vi "DAQ_SampleLoop.vi"(0 "reference in":refnum<class "NI_DAQ.lvclass">, 5 "error in (no error)":errorcluster) -> (14 "reference out":refnum<class "NI_DAQ.lvclass">, 15 "RealTimeValue":dbl[](array[numeric]), 19 "error out":errorcluster)   [LabVIEW 2020, in "DAQ.lvlib" / "NI_DAQ.lvclass"]
uses:
  NI_DAQ.lvclass
  D:/BingoGithub/DAQ_V000.04/DAQ_Module/DAQ_Base_class/DAQ_Base.lvclass
  DAQ_Base_class/DAQ_Base.lvclass
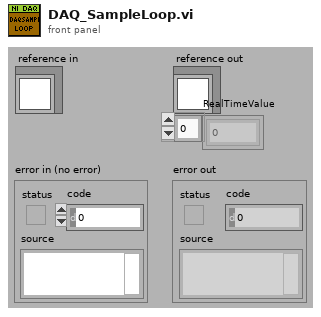
[diagram p1: front panel]
types:
  T1 = typedef "DAQ.lvlib/DAQ_Base.lvclass/ObjectAttributesRef.ctl" = refnum<data-value>
  T2 = typedef "DAQ.lvlib/DAQ_Base.lvclass/ObjectAttributes.ctl" = cluster{"MyAttribute":dbl, "RootPath":path, "DAQSettings":T3, "DaqCollector":cluster{"CollectDataQueue":refnum<queue>, "ArryDataCollectorChannel":T9[], "RealTimeValues":dbl[]}, "CollectorChannelEnable":bool[]}
  T3 = typedef "DAQ.lvlib/DAQ_Base.lvclass/DAQSettings.ctl" = cluster{"SampleSettings":T4, "AI_ChannelSettings":T5, "AO_ChannelSettings":T7, "Cnt_ChannelSettings":T8}
  T4 = typedef "DAQ.lvlib/DAQ_Base.lvclass/SampleSettings.ctl" = cluster{"samples per channel":i32, "SampleRate":dbl, "TansMaxLength":dbl, "ReadTimeOut":dbl, "时钟源":tag}
  T5 = typedef "DAQ.lvlib/DAQ_Base.lvclass/AI_ChannelSettings.ctl" = cluster{"AI_SettingsArry":cluster{"DeviceName":tag, "physical channels":tag, "AssignName":string, "输入信号类型":T6, "Max_value":dbl, "Min_value":dbl, "单位":i32, "shunt resistor location":i32, "external shunt resistor value":dbl, "标定系数":cluster{"Scale":dbl, "Offset":dbl}}[]}
  T6 = typedef "AI信号类型.ctl" = i32
  T7 = typedef "DAQ.lvlib/DAQ_Base.lvclass/AO_ChannelSettings.ctl" = cluster{"布尔":bool}
  T8 = typedef "DAQ.lvlib/DAQ_Base.lvclass/Cnt_ChannelSettings.ctl" = cluster{"Cnt_ChannelSettings":cluster{"类型":enum16{"Linear", "Rotate"}, "CounterNbr":tag, "AssignName":string, "单位":u16, "decoding type":u16, "PPR_DistancePerPulse":dbl, "Initial Position ":dbl, "z index enable":bool, "z index phase":i32, "source":tag}[]}
  T9 = typedef "DAQ.lvlib/DAQ_Base.lvclass/DataCollector.ctl" = cluster{"DataCollectArry":dbl[][], "Update":bool}
  T10 = cluster{"DeviceName":tag, "physical channels":tag, "AssignName":string, "输入信号类型":T6, "Max_value":dbl, "Min_value":dbl, "单位":i32, "shunt resistor location":i32, "external shunt resistor value":dbl, "标定系数":cluster{"Scale":dbl, "Offset":dbl}}[]
  T11 = typedef "DAQ.lvlib/NI_DAQ.lvclass/ObjectAttributes.ctl" = cluster{"MyAttribute":dbl, "DAQ_AI_task_out":refnum<k21>, "counter_task_out":refnum<k21>[]}
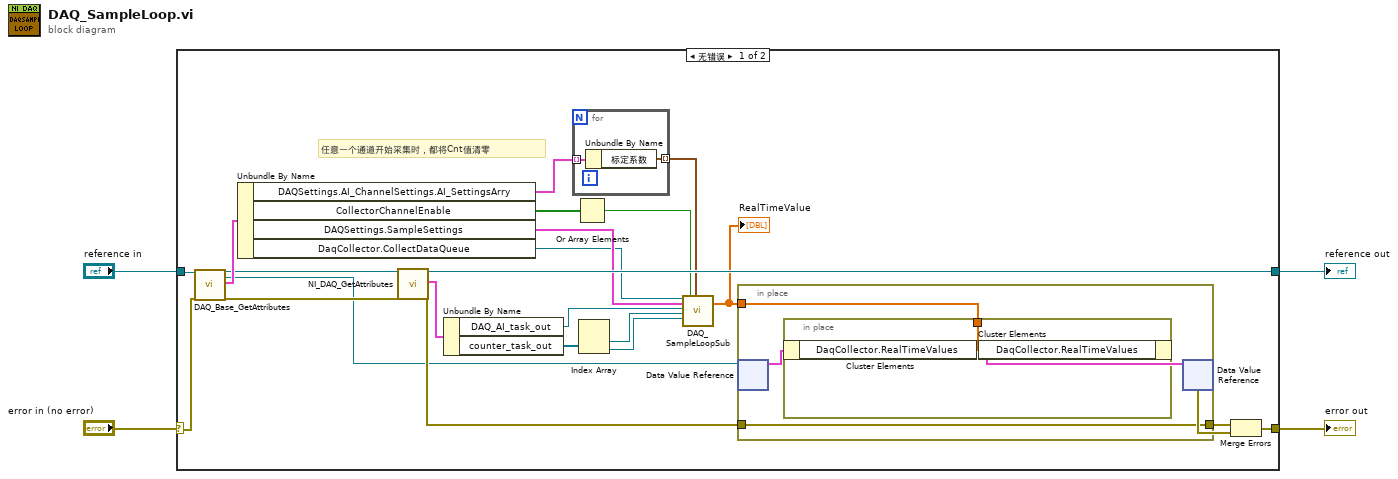
[diagram p0: block diagram]
diagram:
  n1 = case shown="无错误" "error in (no error)" {
    selector: "error in (no error)" -> [w11 w36]
    tunnel: [w27 w36] -> w3
    tunnel: [w26 w35] -> w1
    tunnel: "reference in" -> [w16 w35]
    frame No Error {
      # "任意一个通道开始采集时，都将Cnt值清零"
      n2 = call "DAQ_Base_GetAttributes.vi"("reference in"=w16, "error in (no error)"=w11) -> ("reference out"=w13:refnum<class "NI_DAQ.lvclass">, "attributes ref"=w8:T1, "attributes"=w15:T2, "error out"=w12:errorcluster)  [unwired: 14 in]
      n3 = Unbundle By Name(w15) -> ("DAQSettings.AI_ChannelSettings.AI_SettingsArry"=w6:T10, "CollectorChannelEnable"=w10:bool[], "DAQSettings.SampleSettings"=w17:T4, "DaqCollector.CollectDataQueue"=w14:refnum<queue>)
      n4 = call "NI_DAQ_GetAttributes.vi"("reference in"=w13, "error in (no error)"=w12) -> ("reference out"=w26:refnum<class "NI_DAQ.lvclass">, "attributes"=w24:T11, "error out"=w25:errorcluster)  [unwired: 14 in, 1 out]
      n5 = Unbundle By Name(w24) -> ("DAQ_AI_task_out"=w21:refnum<k21>, "counter_task_out"=w20:refnum<k21>[])
      n6 = for {
        tunnel: w6 -> [w29] mode=indexing
        tunnel: [w28] -> w5 mode=indexing
        n7 = Unbundle By Name(w29) -> ("标定系数"=w28:cluster{"Scale":dbl, "Offset":dbl})
      }
      n8 = Or Array Elements(Boolean array=w10) -> (logical OR=w9:bool)
      n9 = Index Array(array=w20) -> (element #1=w19:refnum<k21>, element #2=w18:refnum<k21>)  [unwired: 2 in]
      n10 = call "DAQ_SampleLoopSub.vi"("DAQ_collectQueue"=w14, "SampleSettings"=w17, "AI_task"=w21, "CntTask 1"=w19, "CntTask 2"=w18, "ClearCnt"=w9, "sensor_arrtribute"=w5) -> ("RealTimeValue"=w7:dbl[])  [unwired: 12 in]
      "RealTimeValue" <- w7
      n11 = in-place {
        in-place-border: w25 -> [w31]
        in-place-border: [w31] -> w23
        in-place-border: w7 -> [w30]
        n12 = in-place-dvr #1(w8) -> (w32:T2)  [unwired: 1 out]
        n13 = in-place {
          in-place-border: w30 -> [w34]
          n14 = in-place-cluster #2(w32) -> ()  [unwired: 1 out]
          n15 = in-place-cluster #2("DaqCollector.RealTimeValues"=w34) -> (w33:T2)
        }
        n16 = in-place-dvr #1(w33) -> (w22:errorcluster)  [unwired: 1 out]
      }
      n17 = Merge Errors(w23, w22) -> (w27:errorcluster)
    }
    frame Error {
    }
  }
  "error out" <- w3
  "reference out" <- w1
